vi "IMAQ-MWT DMD Intensity Calibration (HOST).vi"() -> ()   [LabVIEW 2015]
uses:
  Modules/Common/Controls (HOST)/Image Size.ctl
  Modules/Common/Controls (HOST)/REF.ctl
  Modules/Common/Controls (HOST)/Image Queue Bundle.ctl
  Modules/Common/Controls (HOST)/Data to Disk Bundle.ctl
  Modules/Common/Controls (HOST)/FPGA REF (MWT).ctl
  Modules/Common/Controls (HOST)/Main States.ctl
  Modules/Common/Controls (HOST)/IMAQ Parameters.ctl
  Modules/Common/Controls (HOST)/File REF.ctl
  <vilib>/vision/Avi.llb/IMAQ AVI2 Refnum.ctl
  Modules/Common/Controls (HOST)/Experiment Mode.ctl
  <vilib>/Utility/error.llb/Error Cluster From Error Code.vi
  <vilib>/rvi/errors/niLvFpgaAdjustHostInterfaceError.vi
  <vilib>/FPGAPlugInAG/Dynamic/niLvFpga_Close_Dynamic.vi
  <vilib>/imath/engines/lvmath2/RunTimeEngine/Managers/WorkSpace/UID Generator.vi
  <vilib>/imath/engines/lvmath2/RunTimeEngine/RunTimeType/NIMS_RunTimeType_From StrictType (excl LVString).vi
  <instcachedir>/0/NIMS_RunTimeType_From StrictType (excl LVString)_EB1C38A9BC5048DA9ABDA8F781E54D21.lvgen/NIMS_RunTimeType_From StrictType (excl LVString)_EB1C38A9BC5048DA9ABDA8F781E54D21_031.vi
  <vilib>/imath/engines/lvmath2/RunTimeEngine/Struct/NIMS_StructSetField.vi
  <vilib>/imath/engines/lvmath2/RunTimeEngine/Struct/NIMS_StructGetField.vi
  <vilib>/imath/engines/lvmath2/RunTimeEngine/RunTimeType/NIMS_RunTimeType_To Numeric.vi
  <instcachedir>/0/NIMS_RunTimeType_To Numeric_B134FEC7BFC54ED5998F4CFD2EE98288.lvgen/NIMS_RunTimeType_To Numeric_B134FEC7BFC54ED5998F4CFD2EE98288_008.vi
  <instcachedir>/0/NIMS_RunTimeType_From StrictType (excl LVString)_EB1C38A9BC5048DA9ABDA8F781E54D21.lvgen/NIMS_RunTimeType_From StrictType (excl LVString)_EB1C38A9BC5048DA9ABDA8F781E54D21_000.vi
  <vilib>/imath/engines/lvmath2/RunTimeEngine/LocalVariableDefStatement/MC_LocalVariableDefStatement_Display.vi
  <vilib>/imath/engines/lvmath2/RunTimeEngine/Managers/SymbolTable/Clear UID.vi
  <vilib>/imath/engines/lvmath2/RunTimeEngine/NodeEndStatement/NIMS_NodeEndStatement_Output.vi
  <instcachedir>/0/NIMS_NodeEndStatement_Output_53EC0D466D134D7ABD903AC30B43404B.lvgen/NIMS_NodeEndStatement_Output_53EC0D466D134D7ABD903AC30B43404B_001.vi
  <vilib>/imath/engines/lvmath2/RunTimeEngine/ErrorHandling/NIMS_Finalize Error.vi
  <vilib>/Utility/file.llb/Write Delimited Spreadsheet (DBL).vi
  <vilib>/rvi/interface/nirviReadWriteControl/nirviReadWriteControl.xnode
  <vilib>/rvi/interface/nirviCloseFPGA/nirviCloseFPGA.xnode
  NiFpgaLv.dll
  <vilib>/rvi/interface/Simulation/niFpgaSimulationCallBeginRW.vi
  <vilib>/imath/engines/lvmath2/RunTimeEngine/Managers/SymbolTable/NIMS_WorkSpace.lvlib
panel:
  in  "DMD #":enum16{"DMD1", "DMD2"}(ring)
  in  "Rows Complete":i32
  in  "Int Coeff":bool
  in  "Intensity (mW/cm2)":dbl[][](array[numeric])
  in  "Save Int":bool
  in  "Measured Intensity (uW/cm2)":dbl format="%.2f"
  in  "Current Measurement Spot":cluster{"Rows":u32, "Columns":u32}={"Rows"=1, "Columns"=1} {"Columns" min=1 step=1; "Rows" min=1 step=1}
  out "Total Number of Calibration Points":u32
  in  "Number of Calibration Points":cluster{"Rows":u32, "Columns":u32}={"Rows"=4, "Columns"=4}
  in  "Image Size":T1={"Height"=3072, "Width"=3200}
  out "Frame Rate":u32
  out "Frame #":u32
  in  "Stop Button":bool
  in  "Go":bool
  in  "Height":i32=100
  in  "Width":i32=100
  in  "Y":i32=334
  in  "X":i32=462
  out "Exp. Status":string="Camera Connected"
  out "REF":T2
  out "Command Q":refnum<queue>
  out "Display":T5(plugin-control)
  out "Stopped?":bool
  # "IMAQ - DMD Intensity Calibration"
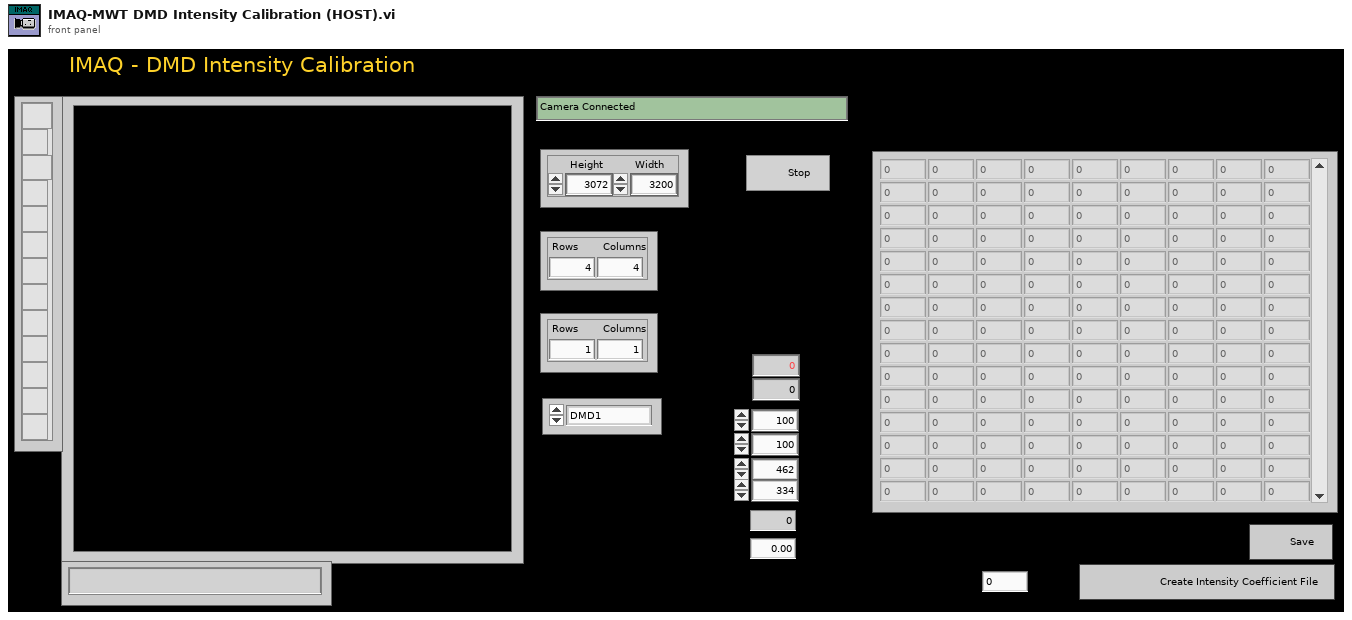
[diagram p1: front panel]
types:
  T1 = typedef "Image Size.ctl" = cluster{"Height":u16, "Width":u16}
  T2 = typedef "REF.ctl" = cluster{"Queue REF":T3, "FPGA REF (MWT)":T4}
  T3 = typedef "Image Queue Bundle.ctl" = cluster{"Disk Image":refnum<queue>, "Image Blocks":refnum<queue>, "Display Image":refnum<queue>, "BG Image":refnum<queue>, "Tag Image":refnum<queue>}
  T4 = typedef "FPGA REF (MWT).ctl" = refnum<k20>
  T5 = typedef "IMAQ Image.ctl" = refnum<image>
  T6 = enum8{"Enabled", "Disabled", "Disabled and Grayed Out"}
  T7 = typedef "Main States.ctl" = enum16{"Open FPGA", "Initialize", "Preview", "Acquire Images", "STOP"}
  T8 = typedef "Experiment Mode.ctl" = enum16{"Live", "Replay"}
  T9 = typedef "IMAQ Parameters.ctl" = cluster{"File REF":T10, "Frame Data":cluster{"Width":u32, "Height":u32, "Frames Per Second":u32, "Codec":string}, "File Type":string, "Experiment Mode":T8, "Movie File Path":path}
  T10 = typedef "File REF.ctl" = cluster{"AVI REF":T11, "DBDE REF":refnum<file>}
  T11 = typedef "IMAQ AVI2 Refnum.ctl" = refnum<k20>
  T12 = typedef "Data to Disk Bundle.ctl" = cluster{"Frame Number":u64, "Time Stamp (us)":u64, "Image Data":u64[], "Contour":u32[], "Raw Image REF":refnum<data-value>, "Block Image REF":refnum<data-value>, "Block Box":u64[], "SPINE":u32[], "HT Angle":u64[], "Block Position":u64[], "SPINE Count":u32[], "Contour Count":u32[], "SPINE DIR":u8[]}
  T13 = typedef "DMD 2 Calibration Parameters.ctl" = cluster{"xm1":dbl, "ym1":dbl, "xm2":dbl, "ym2":dbl, "xoff":dbl, "yoff":dbl}
  T14 = typedef "DMD 1 Calibration Parameters.ctl" = cluster{"xm1":dbl, "ym1":dbl, "xm2":dbl, "ym2":dbl, "xoff":dbl, "yoff":dbl}
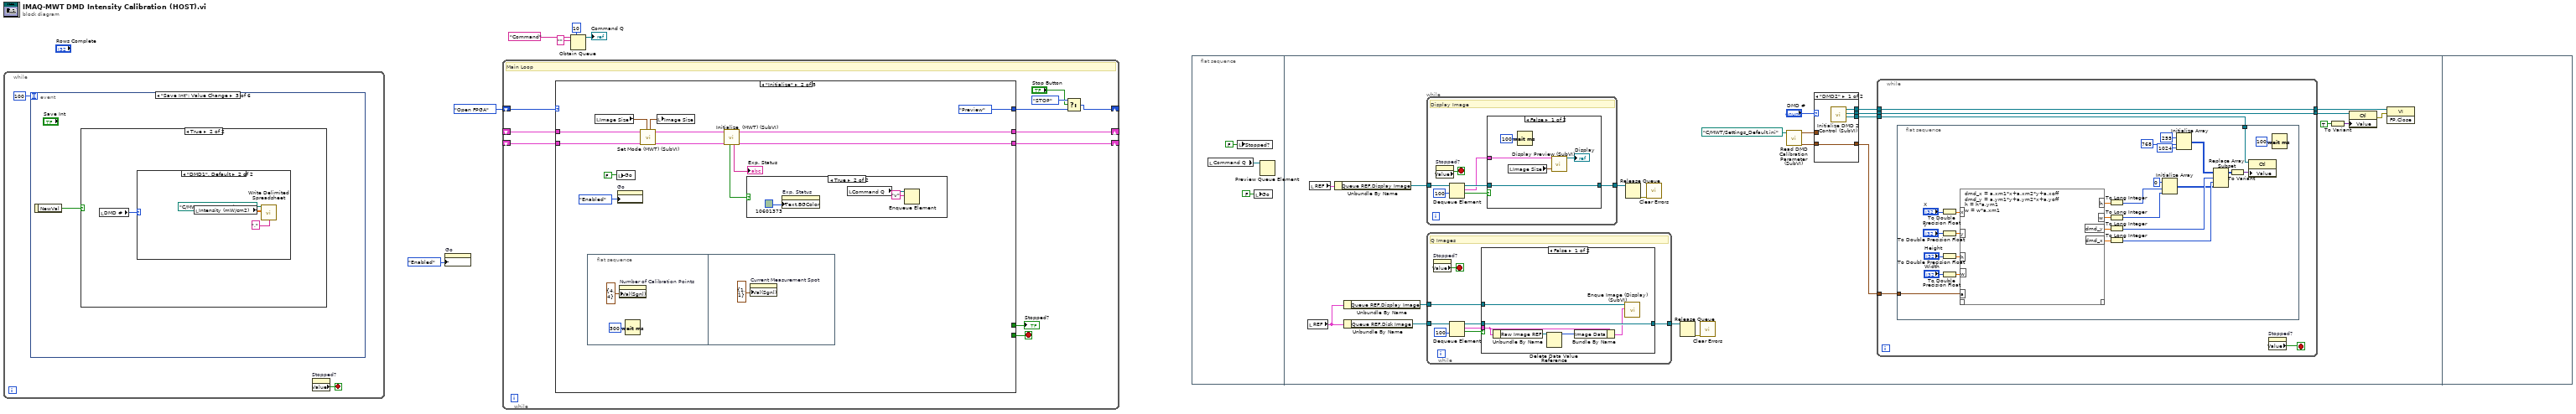
[diagram p0: block diagram]
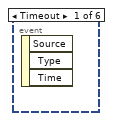
[diagram p2: hidden frame]
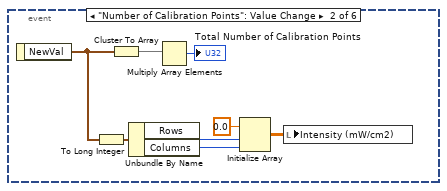
[diagram p3: hidden frame]
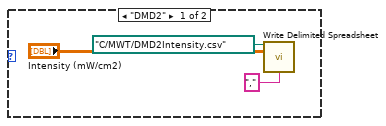
[diagram p5: hidden frame]
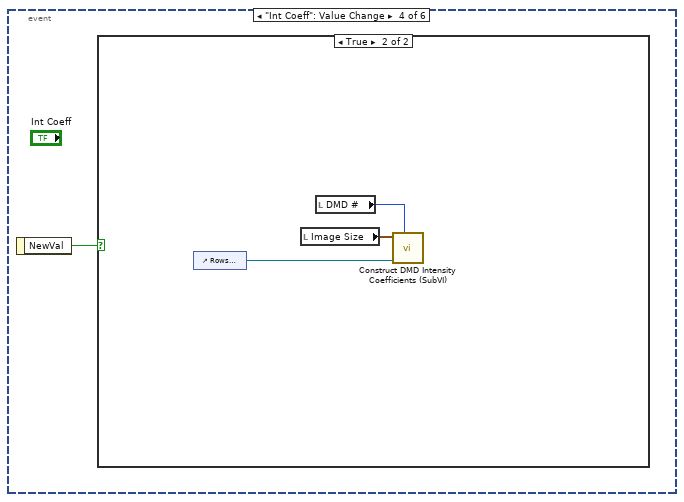
[diagram p6: hidden frame]
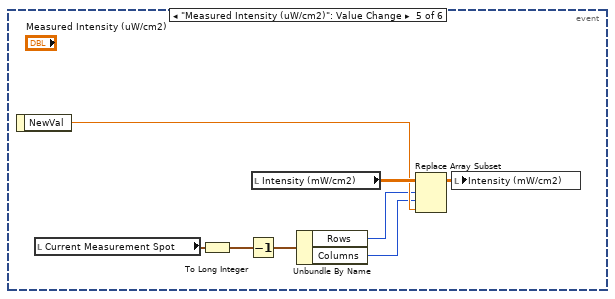
[diagram p8: hidden frame]
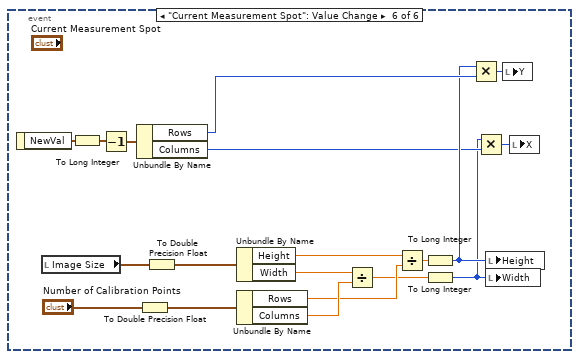
[diagram p9: hidden frame]
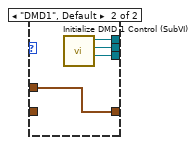
[diagram p10: hidden frame]
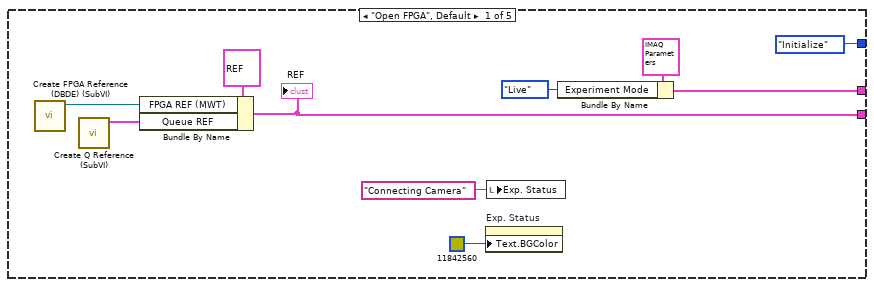
[diagram p13: hidden frame]
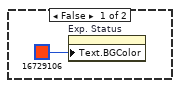
[diagram p14: hidden frame]
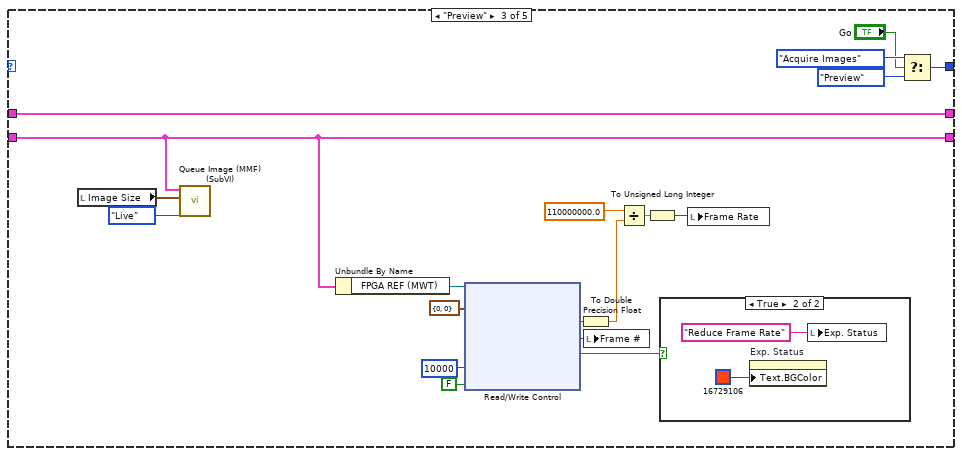
[diagram p15: hidden frame]
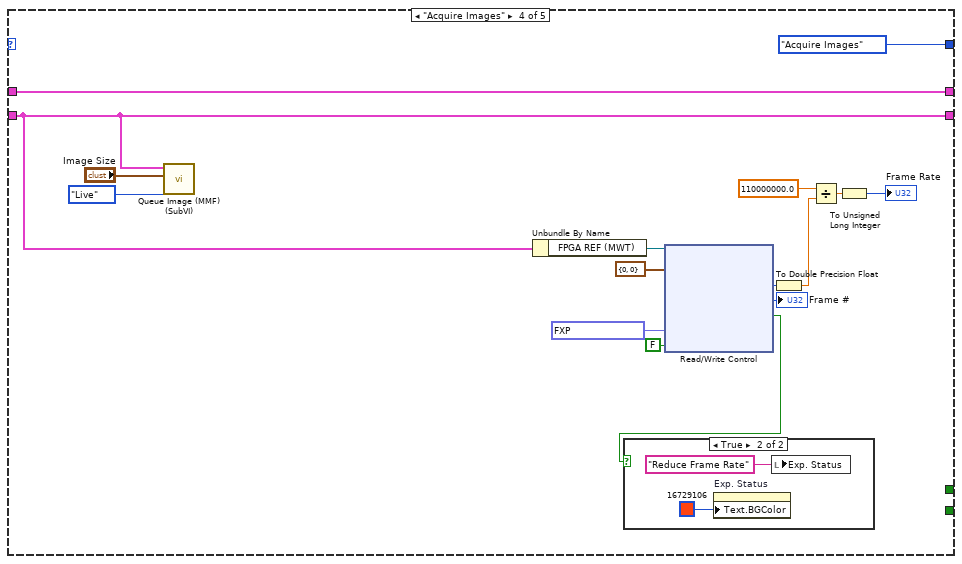
[diagram p17: hidden frame]
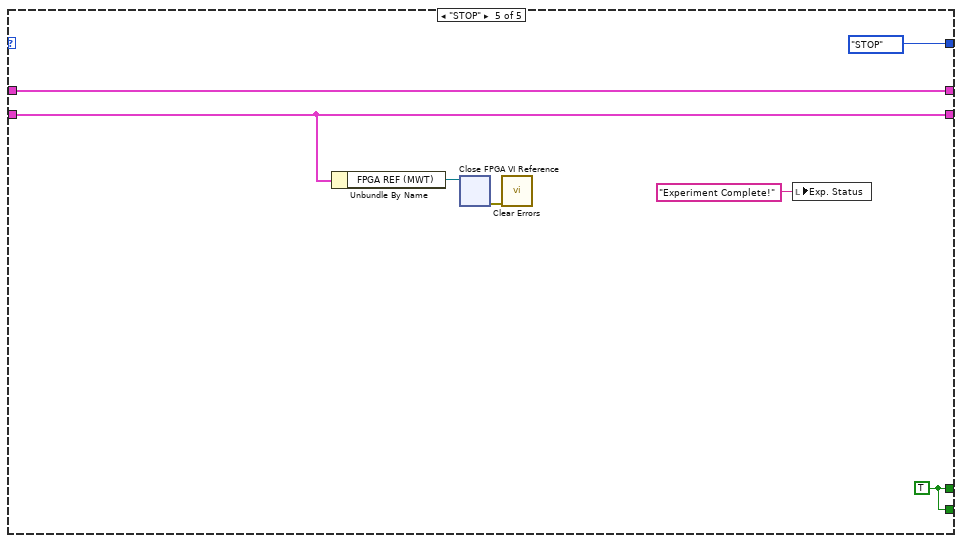
[diagram p19: hidden frame]
diagram:
  n1 = while {
    stop <- w8 stop-if-true
    n2 = event shown="[2] \"Save Int\": Value Change" {
      selector: _ -> [_ _ _ _ _ _]
      dyn-events: _ -> [_ _ _ _ _ _]
      timeout: 100 -> [_ _ _ _ _ _]
      event Timeout {
        n3 = event-data() -> ()  [unwired: 1 in, 3 out]
      }
      event "Number of Calibration Points": Value Change {
        n4 = event-data() -> ("NewVal"=w14:cluster{"Rows":u32, "Columns":u32})  [unwired: 1 in]
        n5 = To Long Integer(number=w14) -> (32bit integer=w10:cluster{"Rows":i32, "Columns":i32})
        n6 = Cluster To Array(cluster=w14) -> (array=w15:u32[])
        n7 = Unbundle By Name(w10) -> ("Rows"=w13:i32, "Columns"=w12:i32)
        n8 = Multiply Array Elements(1:w15) -> (0:→"Total Number of Calibration Points":u32)
        n9 = Initialize Array(0.0 ("element"), w13, w12) -> (w9:dbl[][])
        n10 = local write "Intensity (mW/cm2)"(w9) -> ()
      }
      event "Save Int": Value Change {
        n11 = event-data() -> ("NewVal"=w17:bool)  [unwired: 1 in]
        n12 = case shown="True" w17 {
          frame False {
          }
          frame True {
            n13 = local read "DMD #"() -> (w18:enum16{"DMD1", "DMD2"})
            n14 = case shown="\"DMD1\", Default" w18 {
              frame "DMD2" {
                n15 = call-poly <vilib>:"Write Delimited Spreadsheet.vi"("file path (dialog if empty)"=path "C:/MWT/DMD2Intensity.csv", "2D data"="Intensity (mW/cm2)", "delimiter (\\t)"="," ("delimiter (\\t)")) -> ()  [unwired: 11 in, 2 out]
              }
              frame "DMD1", Default {
                n16 = local read "Intensity (mW/cm2)"() -> (w22:dbl[][])
                n17 = call-poly <vilib>:"Write Delimited Spreadsheet.vi"("file path (dialog if empty)"=path "C:/MWT/DMD1Intensity.csv", "2D data"=w22, "delimiter (\\t)"="," ("delimiter (\\t)")) -> ()  [unwired: 11 in, 2 out]
              }
            }
          }
        }
      }
      event "Int Coeff": Value Change {
        n18 = event-data() -> ("NewVal"=w25:bool)  [unwired: 1 in]
        n19 = case shown="True" w25 {
          frame False {
          }
          frame True {
            n20 = control-ref of="Rows Complete"() -> (w27:refnum<vi>)
            n21 = local read "Image Size"() -> (w28:T1)
            n22 = local read "DMD #"() -> (w26:enum16{"DMD1", "DMD2"})
            n23 = call "Construct DMD Intensity Coefficients (SubVI).vi"("DMD #"=w26, "Number of Rows Processed"=w27, "Image Size in"=w28) -> ()  [unwired: 9 in]
          }
        }
      }
      event "Measured Intensity (uW/cm2)": Value Change {
        n24 = event-data() -> ("NewVal"=w35:dbl)  [unwired: 1 in]
        n25 = local read "Current Measurement Spot"() -> (w34:cluster{"Rows":u32, "Columns":u32})
        n26 = To Long Integer(number=w34) -> (32bit integer=w31:cluster{"Rows":i32, "Columns":i32})
        n27 = Decrement(x=w31) -> (x-1=w29:cluster{"Rows":i32, "Columns":i32})
        n28 = local read "Intensity (mW/cm2)"() -> (w36:dbl[][])
        n29 = Unbundle By Name(w29) -> ("Rows"=w33:i32, "Columns"=w32:i32)
        n30 = Replace Array Subset(array=w36, new element=w35, index (row)=w33, index (col)=w32) -> (w30:dbl[][])
        n31 = local write "Intensity (mW/cm2)"(w30) -> ()
      }
      event "Current Measurement Spot": Value Change {
        n32 = event-data() -> ("NewVal"=w45:cluster{"Rows":u32, "Columns":u32})  [unwired: 1 in]
        n33 = local read "Image Size"() -> (w55:T1)
        n34 = To Long Integer(number=w45) -> (32bit integer=w41:cluster{"Rows":i32, "Columns":i32})
        n35 = Decrement(x=w41) -> (x-1=w44:cluster{"Rows":i32, "Columns":i32})
        n36 = Unbundle By Name(w44) -> ("Rows"=w43:i32, "Columns"=w38:i32)
        n37 = To Double Precision Float(number="Number of Calibration Points") -> (double precision float=w52:cluster{"Rows":dbl, "Columns":dbl})
        n38 = To Double Precision Float(number=w55) -> (double precision float=w53:cluster{"Height":dbl, "Width":dbl})
        n39 = Unbundle By Name(w53) -> ("Height"=w51:dbl, "Width"=w50:dbl)
        n40 = Unbundle By Name(w52) -> ("Rows"=w48:dbl, "Columns"=w49:dbl)
        n41 = Divide(x=w50, y=w49) -> (x/y=w47:dbl)
        n42 = Divide(x=w51, y=w48) -> (x/y=w46:dbl)
        n43 = To Long Integer(number=w46) -> (32bit integer=w40:i32)
        n44 = To Long Integer(number=w47) -> (32bit integer=w37:i32)
        n45 = Multiply(x=w40, y=w43) -> (x*y=w42:i32)
        n46 = Multiply(x=w37, y=w38) -> (x*y=w39:i32)
        n47 = local write "Height"(w40) -> ()
        n48 = local write "Width"(w37) -> ()
        n49 = local write "Y"(w42) -> ()
        n50 = local write "X"(w39) -> ()
      }
    }
    n51 = property on="Stopped?" class="Bool (strict)"() -> ("Value"=w8:bool)  [unwired: 2 in, 2 out]
  }
  n52 = property on="Go" class="Bool (strict)"("DisabledEnum"=T6."Enabled" ("Disabled")) -> ()  [unwired: 2 in, 2 out]
  n53 = while {
    shift-right: [w65] -> _
    shift-left: _ -> [w64]
    shift-right: [w56] -> _
    shift-left: Main_States."Open FPGA" -> [w66]
    shift-right: [w58] -> _
    shift-left: _ -> [w57]
    stop <- w62 stop-if-true
    # "Main Loop"
    n54 = case shown="\"Initialize\"" w66 {
      tunnel: [w73 w77 w101 w123 w139] -> w65
      tunnel: w64 -> [_ w78 w101 w123 w139]
      tunnel: [Main_States."Initialize" Main_States."Preview" w114 Main_States."Acquire Images" Main_States."STOP"] -> w63
      tunnel: [_ _ _ _ w141] -> w62
      tunnel: [_ _ _ _ w141] -> w61
      tunnel: [w68 w82 w107 w124 w138] -> w58
      tunnel: w57 -> [_ w88 w107 w124 w138]
      frame "Open FPGA", Default {
        n55 = call "Create FPGA Reference (DBDE) (SubVI).vi"() -> ("FPGA REF (MWT)"=w75:T4)  [unwired: 11 in]
        n56 = call "Create Q Reference (SubVI).vi"() -> ("Image Queue"=w74:T3)  [unwired: 11 in]
        n57 = Bundle By Name(cluster=T2 {"Queue REF"={"Disk Image"=refnum, "Image Blocks"=refnum, "Display Image"=refnum, "BG Image"=refnum, "Tag Image"=refnum}, "FPGA REF (MWT)"=refnum}, "FPGA REF (MWT)"=w75, "Queue REF"=w74) -> (w73:T2)
        "REF" <- w73
        n58 = property on="Exp. Status" class="Str"("Text.BGColor"=u32 11842560) -> ()  [unwired: 2 in, 2 out]
        n59 = local write "Exp. Status"("Connecting Camera" ("Exp. Status")) -> ()
        n60 = Bundle By Name(cluster=T9 {"File REF"={"AVI REF"=refnum, "DBDE REF"=refnum}, "Frame Data"={"Width"=0, "Height"=0, "Frames Per Second"=0, "Codec"=""}, "File Type"="", "Experiment Mode"=enum."Live", "Movie File Path"=path "D:/Movies Formatted on November 5th 2015/Clip (2) Formatted.raw"} ("Movie File Property"), "Experiment Mode"=Experiment_Mode."Live") -> (w68:T9)
      }
      frame "Initialize" {
        n61 = flat-sequence {
          frame #0 {
            n62 = property on="Number of Calibration Points" class="Clust (strict)"("Val(Sgnl)"=cluster{"Rows":u32, "Columns":u32} {"Rows"=4, "Columns"=4} ("Value (Signaling)")) -> ()  [unwired: 2 in, 2 out]
            n63 = Wait (ms)(milliseconds to wait=u32 300) -> ()  [unwired: 1 out]
          }
          frame #1 {
            n64 = property on="Current Measurement Spot" class="Clust (strict)"("Val(Sgnl)"=cluster{"Rows":u32, "Columns":u32} {"Rows"=1, "Columns"=1} ("Value (Signaling)")) -> ()  [unwired: 2 in, 2 out]
          }
        }
        n65 = local read "Image Size"() -> (w80:T1)
        n66 = local write "Go"(FALSE ("Go")) -> ()
        n67 = property on="Go" class="Bool (strict)"("DisabledEnum"=T6."Enabled" ("Disabled")) -> ()  [unwired: 2 in, 2 out]
        n68 = call "Set Mode (MWT) (SubVI).vi"("Image Size In"=w80, "REF IN"=w78, "Parameters In"=w88) -> ("REF OUT"=w81:T2, "Parameters Out"=w83:T9, "Image Size Out"=w79:T1)  [unwired: 6 in]
        n69 = local write "Image Size"(w79) -> ()
        n70 = call "Initialize  (MWT) (SubVI).vi"("REF IN"=w81, "Parameters In"=w83) -> ("REF OUT"=w77:T2, "Parameters Out"=w82:T9, "Exp. Status"=→"Exp. Status":string, "OK?"=w85:bool)  [unwired: 6 in]
        n71 = case shown="True" w85 {
          frame False {
            n72 = property on="Exp. Status" class="Str"("Text.BGColor"=u32 16729106) -> ()  [unwired: 2 in, 2 out]
          }
          frame True {
            n73 = property on="Exp. Status" class="Str"("Text.BGColor"=u32 10601373) -> ()  [unwired: 2 in, 2 out]
            n74 = local read "Command Q"() -> (w95:refnum<queue>)
            n75 = Enqueue Element(queue=w95, element="v") -> ()  [unwired: 2 in, 3 out]
          }
        }
      }
      frame "Preview" {
        n76 = local read "Image Size"() -> (w104:T1)
        n77 = call "Queue Image (MMF) (SubVI).vi"("Experiment Mode"=Experiment_Mode."Live", "Image Size"=w104, "Data Bundle"=w101) -> ()  [unwired: 9 in]
        n78 = Unbundle By Name(w101) -> ("FPGA REF (MWT)"=w110:T4)
        n79 = xnode "Read/Write Control"("FPGA VI Reference In"=w110, "Pixel Intensity"=cluster{"Low":u8, "High":u8} {"Low"=0, "High"=0}, "Clock Cycles Limit"=u32 10000, "Swap Bytes"=FALSE) -> ("Frame Interval"=w112:u32, "Frame #"=w103:u32, "DMA Timeout"=w102:bool)  [unwired: 1 in, 2 out]
        n80 = To Double Precision Float(number=w112) -> (double precision float=w111:dbl)
        n81 = local write "Frame #"(w103) -> ()
        n82 = Divide(x=110000000.0 ("y"), y=w111) -> (x/y=w108:dbl)
        n83 = To Unsigned Long Integer(number=w108) -> (unsigned 32bit integer=w106:u32)
        n84 = case shown="True" w102 {
          frame False {
          }
          frame True {
            n85 = property on="Exp. Status" class="Str"("Text.BGColor"=u32 16729106) -> ()  [unwired: 2 in, 2 out]
            n86 = local write "Exp. Status"("Reduce Frame Rate" ("Exp. Status")) -> ()
          }
        }
        n87 = local write "Frame Rate"(w106) -> ()
        n88 = Select(t=Main_States."Acquire Images", s="Go", f=Main_States."Preview") -> (s? t:f=w114:T7)
      }
      frame "Acquire Images" {
        n89 = call "Queue Image (MMF) (SubVI).vi"("Experiment Mode"=Experiment_Mode."Live", "Image Size"="Image Size", "Data Bundle"=w123) -> ()  [unwired: 9 in]
        n90 = Unbundle By Name(w123) -> ("FPGA REF (MWT)"=w130:T4)
        n91 = xnode "Read/Write Control"("FPGA VI Reference In"=w130, "Pixel Intensity"=cluster{"Low":u8, "High":u8} {"Low"=0, "High"=0}, "Significant Angle"=fxp<+,16,3> 0.0699462890625, "Swap Bytes"=FALSE) -> ("Frame Interval"=w132:u32, "Frame #"=→"Frame #":u32, "DMA Timeout"=w125:bool)  [unwired: 1 in, 2 out]
        n92 = case shown="True" w125 {
          frame False {
          }
          frame True {
            n93 = property on="Exp. Status" class="Str"("Text.BGColor"=u32 16729106) -> ()  [unwired: 2 in, 2 out]
            n94 = local write "Exp. Status"("Reduce Frame Rate" ("Exp. Status")) -> ()
          }
        }
        n95 = To Double Precision Float(number=w132) -> (double precision float=w131:dbl)
        n96 = Divide(x=110000000.0 ("y"), y=w131) -> (x/y=w127:dbl)
        n97 = To Unsigned Long Integer(number=w127) -> (unsigned 32bit integer=→"Frame Rate":u32)
      }
      frame "STOP" {
        w141 = TRUE
        n98 = Unbundle By Name(w139) -> ("FPGA REF (MWT)"=w140:T4)
        n99 = xnode "Close FPGA VI Reference"("FPGA VI Reference In"=w140) -> ("error out"=w136:errorcluster)  [unwired: 1 in]
        n100 = call <vilib>:"Clear Errors.vi"("error in (no error)"=w136) -> ()  [unwired: 5 in, 2 out]
        n101 = local write "Exp. Status"("Experiment Complete!" ("Exp. Status")) -> ()
      }
    }
    "Stopped?" <- w61
    n102 = Select(t=Main_States."STOP", s="Stop Button", f=w63) -> (s? t:f=w56:T7)
  }
  n103 = Obtain Queue(max queue size (-1, unlimited)=10, name (unnamed)="Command", element data type="" ("name (unnamed)")) -> (queue out=→"Command Q":refnum<queue>)  [unwired: 2 in, 2 out]
  n104 = flat-sequence {
    frame #0 {
      n105 = local read "Command Q"() -> (w145:refnum<queue>)
      n106 = local write "Stopped?"(FALSE ("Stopped?")) -> ()
      n107 = local write "Go"(FALSE ("Go")) -> ()
      n108 = Preview Queue Element(queue=w145) -> ()  [unwired: 2 in, 4 out]
    }
    frame #1 {
      n109 = local read "REF"() -> (w161:T2)
      n110 = local read "REF"() -> (w166:T2)
      n111 = Unbundle By Name(w166) -> ("Queue REF.Display Image"=w165:refnum<queue>)
      n112 = Unbundle By Name(w161) -> ("Queue REF.Display Image"=w162:refnum<queue>)
      n113 = Unbundle By Name(w161) -> ("Queue REF.Disk Image"=w163:refnum<queue>)
      n114 = while {
        tunnel: [w392] -> w167
        tunnel: w165 -> [w391]
        stop <- w389 stop-if-true
        # "Display Image"
        n115 = property on="Stopped?" class="Bool (strict)"() -> ("Value"=w389:bool)  [unwired: 2 in, 2 out]
        n116 = Dequeue Element(queue=w391, timeout in ms (-1)=100) -> (queue out=w393:refnum<queue>, element=w390:T12, timed out?=w394:bool)  [unwired: 1 in, 1 out]
        n117 = case shown="False" w394 {
          tunnel: w393 -> [w400 w401]
          tunnel: [w400 w401] -> w392
          tunnel: w390 -> [w399 _]
          frame False {
            n118 = local read "Image Size"() -> (w397:T1)
            n119 = Wait (ms)(milliseconds to wait=u32 100) -> ()  [unwired: 1 out]
            n120 = call "Display Preview (SubVI).vi"("Display Data"=w399, "Image Size"=w397) -> ("Image Out"=→"Display":T5)  [unwired: 17 in]
          }
          frame True {
          }
        }
      }
      n121 = while {
        tunnel: [w380] -> w164
        tunnel: w163 -> [w374]
        tunnel: w162 -> [w379]
        stop <- w375 stop-if-true
        # "Q Images"
        n122 = property on="Stopped?" class="Bool (strict)"() -> ("Value"=w375:bool)  [unwired: 2 in, 2 out]
        n123 = Dequeue Element(queue=w374, timeout in ms (-1)=100) -> (queue out=w377:refnum<queue>, element=w378:T12, timed out?=w376:bool)  [unwired: 1 in, 1 out]
        n124 = case shown="False" w376 {
          tunnel: w377 -> [w387 w388]
          tunnel: [w387 w388] -> w380
          tunnel: w379 -> [w386 _]
          tunnel: w378 -> [w384 _]
          frame False {
            n125 = Unbundle By Name(w384) -> ("Raw Image REF"=w385:refnum<data-value>)
            n126 = Delete Data Value Reference(data value reference=w385) -> (data value=w383:u64[])  [unwired: 1 in, 1 out]
            n127 = Bundle By Name(cluster=w384, "Image Data"=w383) -> (w382:T12)
            n128 = call "Enque Image (Display) (SubVI).vi"("Data Bundle"=w382, "Display Image REF"=w386) -> ()  [unwired: 10 in]
          }
          frame True {
          }
        }
      }
      n129 = Release Queue(queue=w167) -> (error out=w160:errorcluster)  [unwired: 2 in, 2 out]
      n130 = call <vilib>:"Clear Errors.vi"("error in (no error)"=w160) -> ()  [unwired: 5 in, 2 out]
      n131 = Release Queue(queue=w164) -> (error out=w159:errorcluster)  [unwired: 2 in, 2 out]
      n132 = call <vilib>:"Clear Errors.vi"("error in (no error)"=w159) -> ()  [unwired: 5 in, 2 out]
      n133 = call "Read DMD Calibration Parameter (SubVI).vi"("Settings File Name"=path "C:/MWT/Settings_Default.ini") -> ("DMD 2 Calibration Parameters"=w147:T13, "DMD 1 Calibration Parameters"=w148:T14)  [unwired: 9 in]
      n134 = case shown="\"DMD2\"" "DMD #" {
        tunnel: [w171 w175] -> w158
        tunnel: [w170 w174] -> w157
        tunnel: [w169 w173] -> w151
        tunnel: w148 -> [_ w172]
        tunnel: w147 -> [w168 _]
        tunnel: [w168 w172] -> w146
        frame "DMD2" {
          n135 = call "Initialize DMD 2 Control (SubVI).vi"() -> ("DMD IMG REF"=w169:refnum<vi>, "STOP REF"=w170:refnum<vi>, "DMD VI REF"=w171:refnum<vi>)  [unwired: 9 in]
        }
        frame "DMD1", Default {
          n136 = call "Initialize DMD 1 Control (SubVI).vi"() -> ("DMD IMG REF"=w173:refnum<vi>, "STOP REF"=w174:refnum<vi>, "DMD VI REF"=w175:refnum<vi>)  [unwired: 9 in]
        }
      }
      n137 = while {
        tunnel: w158 -> [w178]
        tunnel: w157 -> [w179]
        tunnel: [w179] -> w155
        tunnel: [w178] -> w152
        tunnel: w151 -> [w177]
        tunnel: w146 -> [w176]
        stop <- w180 stop-if-true
        n138 = flat-sequence {
          tunnel: w177 -> [w205]
          tunnel: w176 -> [w200]
          frame #0 {
            n139 = To Double Precision Float(number="X") -> (double precision float=w197:dbl)
            n140 = To Double Precision Float(number="Y") -> (double precision float=w196:dbl)
            n141 = To Double Precision Float(number="Height") -> (double precision float=w186:dbl)
            n142 = To Double Precision Float(number="Width") -> (double precision float=w187:dbl)
            n143 = mathscript code="dmd_x = a.xm1*x+a.xm2*y+a.xoff\ndmd_y = a.ym1*y+a.ym2*x+a.yoff\nh = h*a.ym1\nw = w*a.xm1"("x"=w197, "y"=w196, "a"=w200, "h"=w186, "w"=w187) -> ("dmd_y"=w193:dbl, "dmd_x"=w192:dbl, "h"=w185:dbl, "w"=w184:dbl)  [unwired: 1 in, 1 out]
            n144 = To Long Integer(number=w185) -> (32bit integer=w183:i32)
            n145 = To Long Integer(number=w184) -> (32bit integer=w182:i32)
            n146 = To Long Integer(number=w193) -> (32bit integer=w191:i32)
            n147 = To Long Integer(number=w192) -> (32bit integer=w190:i32)
            n148 = Initialize Array(u8 0 ("element"), w183, w182) -> (w181:u8[][])
            n149 = Initialize Array(u8 255 ("element"), 768 ("dimension size"), 1024 ("dimension size")) -> (w201:u8[][])
            n150 = Replace Array Subset(array=w201, new element=w181, index (row)=w191, index (col)=w190) -> (w207:u8[][])
            n151 = To Variant(anything=w207) -> (Variant=w206:variant)
            n152 = property class="Ctl"(reference=w205, "Value"=w206) -> ()  [unwired: 1 in, 2 out]
            n153 = Wait (ms)(milliseconds to wait=u32 100) -> ()  [unwired: 1 out]
          }
        }
        n154 = property on="Stopped?" class="Bool (strict)"() -> ("Value"=w180:bool)  [unwired: 2 in, 2 out]
      }
      n155 = To Variant(anything=TRUE ("Wait Until Done")) -> (Variant=w156:variant)
      n156 = property class="Ctl"(reference=w155, "Value"=w156) -> (error out=w153:errorcluster)  [unwired: 1 in, 1 out]
      n157 = invoke class="VI" method="FP.Close"(reference=w152, error in=w153) -> ()  [unwired: 1 in, 3 out]
    }
    frame #2 {
    }
  }
